vi "getHWIO_2_acquireEnable.vi"(8 "error in (no error)":errorcluster, 11 "Camera in":refnum<class "Camera.lvclass">) -> (0 "error out":errorcluster, 1 "polarity":u16(ring)=1 items=["high level"=1, "low level"=2], 2 "on":bool=TRUE, 3 "Camera out":refnum<class "Camera.lvclass">)   [LabVIEW 2019, in "Camera.lvclass"]
doc: "Gets HWIO acquire enable polarity and status (enabled / disabled). Generates an error if camera is recording or if HWIO configuration is not supported."
uses:
  Camera.lvclass
  pco.sdk/TimingControl/TimingControl.lvlib
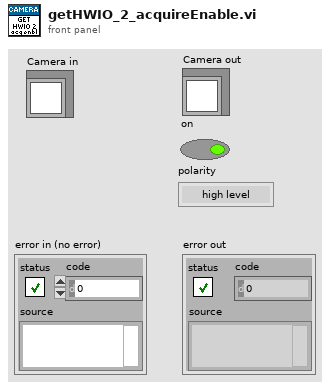
[diagram p1: front panel]
types:
  T1 = cluster{"wSignalNum":u16, "wEnabled":u16, "wType":u16, "wPolarity":u16, "wFilterSetting":u16, "wSelected":u16, "dwParameter":u32[], "dwSignalFunctionality":u32[]}
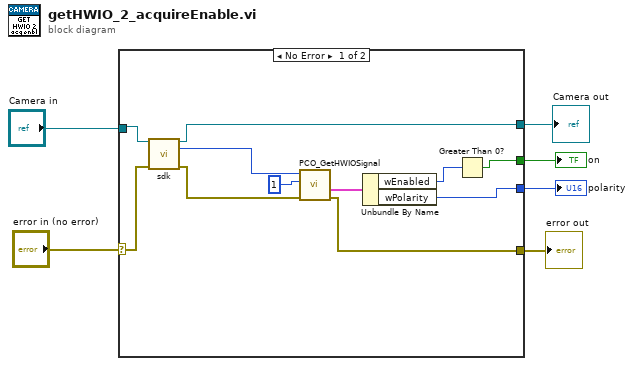
[diagram p0: block diagram]
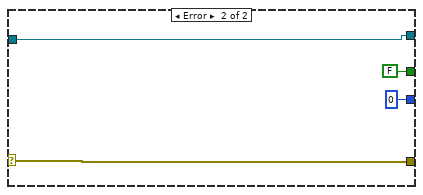
[diagram p2: hidden frame]
diagram:
  n1 = case shown="No Error" "error in (no error)" {
    selector: "error in (no error)" -> [w16 w21]
    tunnel: [w10 w21] -> w3
    tunnel: "Camera in" -> [w17 w20]
    tunnel: [w11 w20] -> w4
    tunnel: [w8 FALSE] -> w2
    tunnel: [w7 u16 0 ("wPolarity")] -> w1
    frame No Error {
      n2 = call-dynamic "sdk.vi"("Camera in"=w17, "error in (no error)"=w16) -> ("Camera out"=w11:refnum<class "Camera.lvclass">, "sdk"=w14:u64, "error out"=w13:errorcluster)  [unwired: 11 in]
      n3 = call "PCO_GetHWIOSignal.vi"("error in (no error)"=w13, "wSignalNum"=u16 1, "ph"=w14) -> ("error out"=w10:errorcluster, "strSignal"=w12:T1)  [unwired: 5 in, 2 out]
      n4 = Unbundle By Name(w12) -> ("wEnabled"=w9:u16, "wPolarity"=w7:u16)
      n5 = Greater Than 0?(x=w9) -> (x > 0?=w8:bool)
    }
    frame Error {
    }
  }
  "Camera out" <- w4
  "error out" <- w3
  "on" <- w2
  "polarity" <- w1
